vi "Temperature Measure 16ch 9213.vi"() -> ()   [LabVIEW 2011]
uses:
  <vilib>/DAQmx/read.llb/DAQmx Read (Analog 1D DBL NChan 1Samp).vi
  <vilib>/DAQmx/create/channels.llb/DAQmx Create Channel (AI-Temperature-Thermocouple).vi
  <vilib>/DAQmx/miscellaneous.llb/DAQmx Fill In Error Info.vi
  C:/Program Files (x86)/National Instruments/LabVIEW 2011/resource/objmgr/daqmx.rc
panel:
  out "Boolean":bool
  in  "Tab Control":enum32{"DISPLAY", "CONFIG"}(tab)
  out "Waveform Chart":T1(graph)={"data[0]"=74.61636698969791, "data[1]"=4164.1284595595835, "data[2]"=4164.1284595595835, "data[3]"=4164.1284595595835, "data[4]"=4164.1284595595835, "data[5]"=4164.1284595595835, "data[6]"=4164.1284595595835, "data[7]"=4164.1284595595835, "data[8]"=4164.1284595595835}
  out "Temperature\nMeasurements":dbl[](array[numeric])=[74.61636698969791, 4164.1284595595835, 4164.1284595595835, 4164.1284595595835, 4164.1284595595835, 4164.1284595595835, 4164.1284595595835, 4164.1284595595835, 4164.1284595595835, 4164.1284595595835, 4164.1284595595835, 4164.1284595595835, 4164.1284595595835, 4164.1284595595835, 4164.1284595595835, 4164.1284595595835] format="%0.2f"
  in  "File Path Input":path
  in  "9213 Name":tag="Dev2"
  out "DAQ Error":errorcluster
  out "Save Error":errorcluster caption="Error Output"
  in  "AI.ADCTimingMode":i32(ring)=10195 items=["High Resolution"=10195, "High Speed"=14712, "Best 50 Hz Rejection"=14713, "Best 60 Hz Rejection"=14714]
  out "daq":i32=1
  out "save":i32=99
  in  "Stop Program":bool=TRUE
  in  "Save Interval (s)":dbl=10.0
  in  "Save (Enable/Signal)":bool
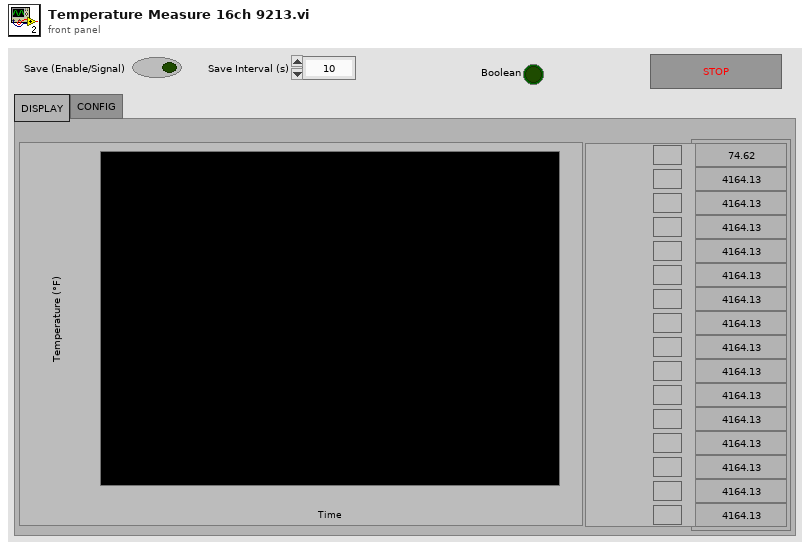
[diagram p1: front panel]
types:
  T1 = cluster{"data[0]":dbl, "data[1]":dbl, "data[2]":dbl, "data[3]":dbl, "data[4]":dbl, "data[5]":dbl, "data[6]":dbl, "data[7]":dbl, "data[8]":dbl}
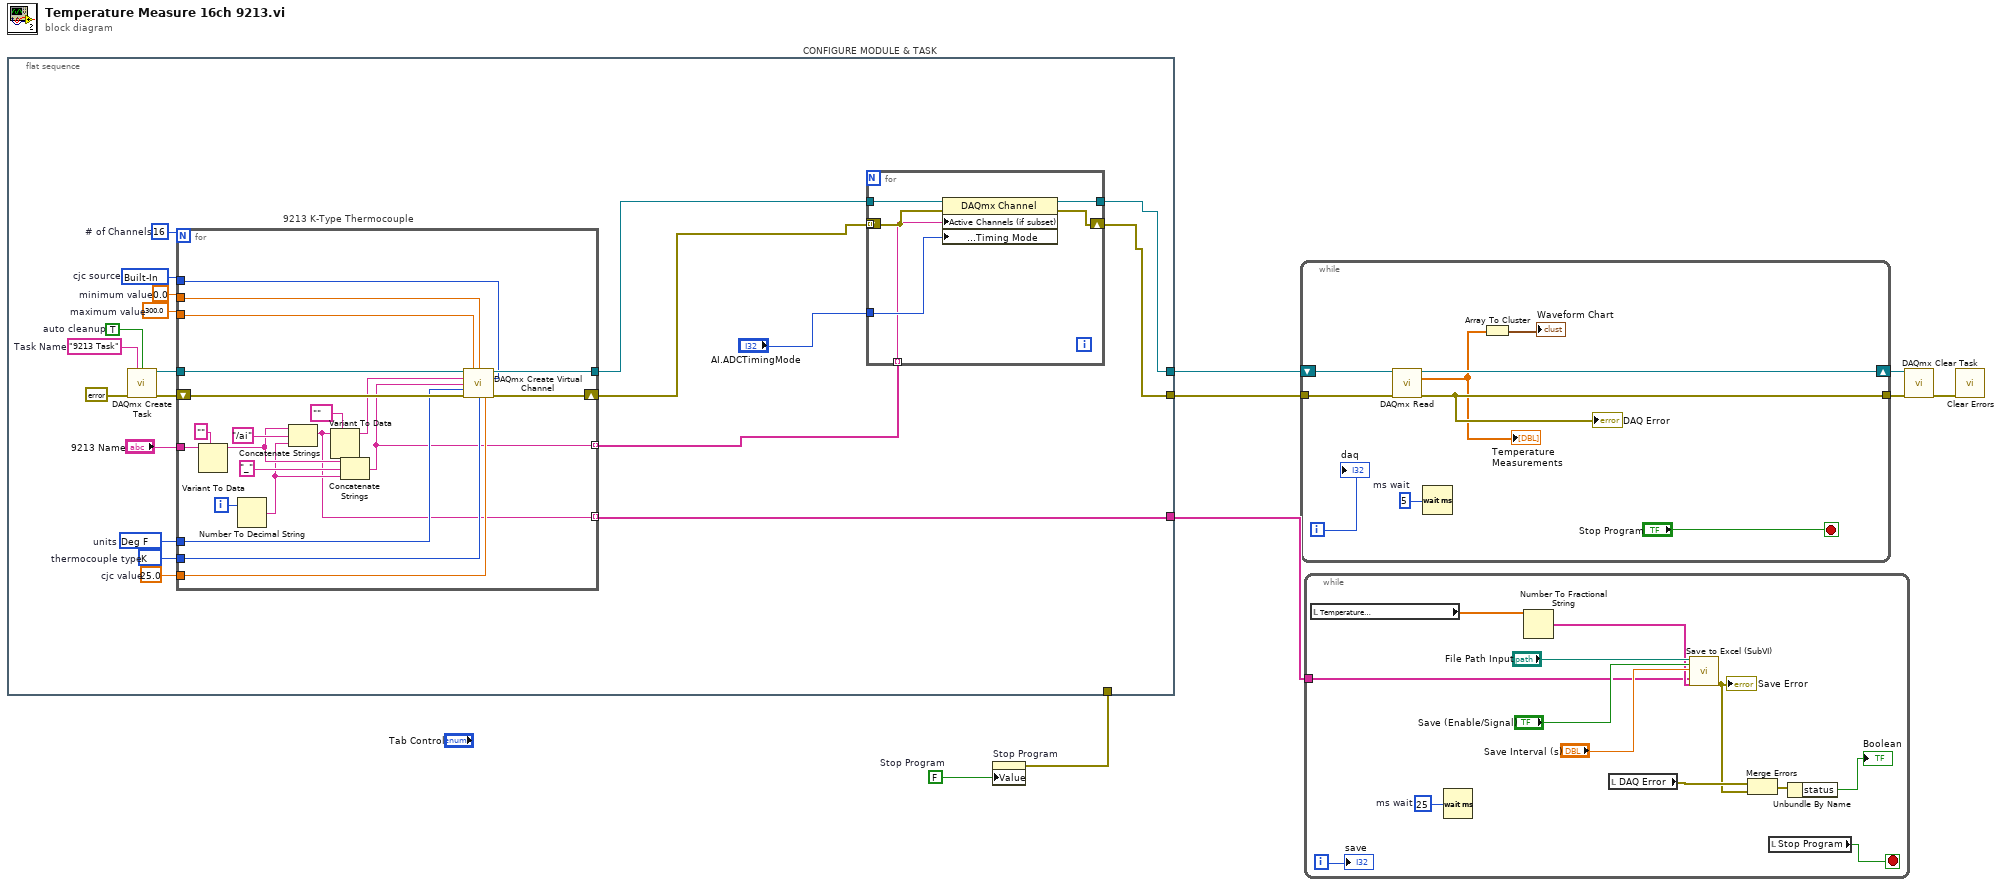
[diagram p0: block diagram]
diagram:
  w2 = FALSE  # Stop Program
  n1 = flat-sequence "CONFIGURE MODULE & TASK" {
    tunnel: [w12] -> w8
    tunnel: [w10] -> w7
    tunnel: [w17] -> w3
    tunnel: w1 -> [_]
    frame #0 {
      w19 = 10144 items=["Deg C"=10143, "Deg F"=10144, "Kelvins"=10325, "Deg R"=10145, "From Custom Scale"=10065]  # units
      w20 = 300.0  # maximum value
      w21 = 0.0  # minimum value
      w22 = 10200 items=["Built-In"=10200, "Constant Value"=10116, "Channel"=10113]  # cjc source
      w15 = 16  # # of Channels
      w23 = 25.0  # cjc value
      w24 = 10073 items=["J"=10072, "K"=10073, "N"=10077, "R"=10082, "S"=10085, "T"=10086, "B"=10047, "E"=10055]  # thermocouple type
      w28 = "9213 Task"  # Task Name
      w26 = TRUE  # auto cleanup
      n2 = call <vilib>:"DAQmx Create Task.vi"("new task name"=w28, "auto cleanup"=w26, "error in"=errorcluster {"status"=FALSE, "code"=0, "source"=""}) -> ("task out"=w27:refnum<k21>, "error out"=w25:errorcluster)  [unwired: 11 in]
      n3 = for "9213 K-Type Thermocouple" {
        N: w15 -> [_]
        tunnel: w27 -> [w55]
        tunnel: [w53] -> w13
        shift-right: [w52] -> w11
        shift-left: w25 -> [w54]
        tunnel: w24 -> [w44]
        tunnel: w23 -> [w43]
        tunnel: w22 -> [w42]
        tunnel: w21 -> [w41]
        tunnel: w20 -> [w40]
        tunnel: w19 -> [w39]
        tunnel: "9213 Name" -> [w38]
        tunnel: [w36] -> w17 mode=indexing
        tunnel: [w35] -> w9 mode=indexing
        i -> [w51]
        n4 = Variant To Data(type="" ("channel name"), Variant=w38) -> (data=w45:string)  [unwired: 1 in, 1 out]
        n5 = Number To Decimal String(number=w51) -> (decimal integer string=w37:string)  [unwired: 1 in]
        n6 = Concatenate Strings(w45, "/ai" ("channel name"), w37) -> (w36:string)
        n7 = Variant To Data(type=tag "" ("physical channels"), Variant=w36) -> (data=w47:tag)  [unwired: 1 in, 1 out]
        n8 = Concatenate Strings(w45, "_" ("channel name"), w37) -> (w35:string)
        n9 = call-poly <vilib>:"DAQmx Create Virtual Channel.vi"("task in"=w55, "maximum value"=w40, "minimum value"=w41, "physical channels"=w47, "cjc source"=w42, "name to assign"=w35, "units"=w39, "error in"=w54, "thermocouple type"=w44, "cjc value"=w43) -> ("task out"=w53:refnum<k21>, "error out"=w52:errorcluster)  [unwired: 4 in]
      }
      n10 = for {
        tunnel: w13 -> [w33]
        shift-right: [w34] -> w10
        shift-left: w11 -> [w31]
        tunnel: [w32] -> w12
        tunnel: "AI.ADCTimingMode" -> [w30]
        tunnel: [w31] -> _ mode=indexing
        tunnel: w9 -> [w29] mode=indexing
        n11 = property class="DAQmx Channel"(reference=w33, error in=w31, "Active Channels (if subset)"=w29, "Analog Input:General Properties:Digitizer/ADC:Timing Mode"=w30) -> (reference out=w32:refnum<k21>, error out=w34:errorcluster)
      }
    }
  }
  n12 = property on="Stop Program" class="Bool (strict)"("Value"=w2) -> (error out=w1:errorcluster)  [unwired: 2 in, 1 out]
  n13 = while {
    shift-right: [w62] -> w6
    shift-left: w8 -> [w64]
    tunnel: w7 -> [w63]
    tunnel: [w59] -> w5
    i -> [w58]
    stop <- "Stop Program" stop-if-true
    w61 = u32 5  # ms wait
    n14 = call-poly <vilib>:"DAQmx Read.vi"("task/channels in"=w64, "error in"=w63) -> ("task out"=w62:refnum<k21>, "data"=w57:dbl[], "error out"=w59:errorcluster)  [unwired: 11 out]
    "Temperature\nMeasurements" <- w57
    "DAQ Error" <- w59
    n15 = Wait (ms)(milliseconds to wait=w61) -> ()  [unwired: 1 out]
    n16 = Array To Cluster(array=w57) -> (cluster=→"Waveform Chart":T1)
    "daq" <- w58
  }
  n17 = while {
    tunnel: w3 -> [w68]
    i -> [w65]
    stop <- w66 stop-if-true
    w74 = u32 25  # ms wait
    n18 = local read "Temperature\nMeasurements"() -> (w69:dbl[])
    n19 = Wait (ms)(milliseconds to wait=w74) -> ()  [unwired: 1 out]
    n20 = Number To Fractional String(number=w69) -> (F-format string=w70:string[])  [unwired: 3 in]
    n21 = local read "DAQ Error"() -> (w75:errorcluster)
    n22 = call "Save to Excel (SubVI).vi"("File Path Input"="File Path Input", "Save (Enable/Signal)"="Save (Enable/Signal)", "Save Interval (s)"="Save Interval (s)", "Column Header Array"=w68, "Data Array (Row)"=w70) -> ("Error Output"=w67:errorcluster)  [unwired: 10 in, 4 out]
    "Save Error" <- w67
    n23 = Merge Errors(w75, w67) -> (w76:errorcluster)
    n24 = local read "Stop Program"() -> (w66:bool)
    n25 = Unbundle By Name(w76) -> ("status"=→"Boolean":bool)
    "save" <- w65
  }
  n26 = call <vilib>:"DAQmx Clear Task.vi"("task in"=w6, "error in"=w5) -> ("error out"=w4:errorcluster)  [unwired: 13 out]
  n27 = call <vilib>:"Clear Errors.vi"("error in (no error)"=w4) -> ()  [unwired: 6 in, 1 out]
